vi "level_control_tank.vi"() -> ()   [LabVIEW 2022 SP3]
uses:
  <vilib>/Instr/_visa.llb/VISA Configure Serial Port (Instr).vi
panel:
  out "Tank":i16(slide) scale=0.0..4000.0
  in  "stop":bool
  in  "Baudrate":string(combo)
  in  "Connect":bool
  in  "VISA resource name":refnum<visa-resource-name>
  in  "Slide":i16(slide) scale=0.0..4000.0
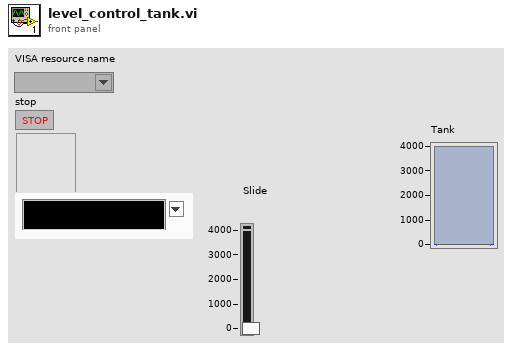
[diagram p1: front panel]
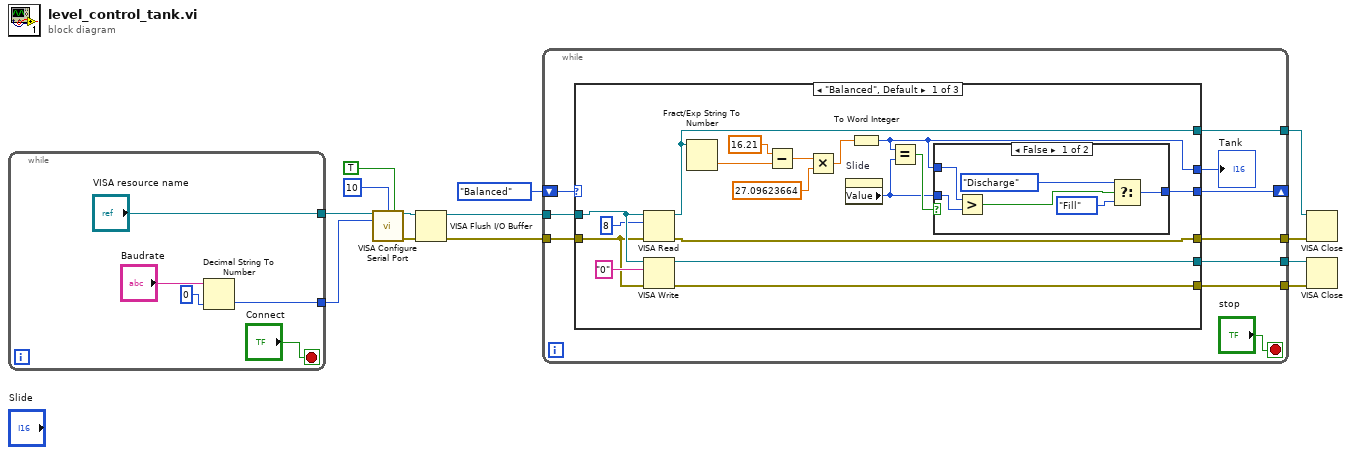
[diagram p0: block diagram]
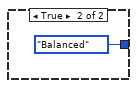
[diagram p2: hidden frame]
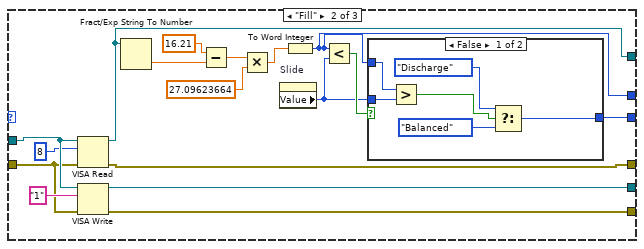
[diagram p3: hidden frame]
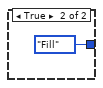
[diagram p4: hidden frame]
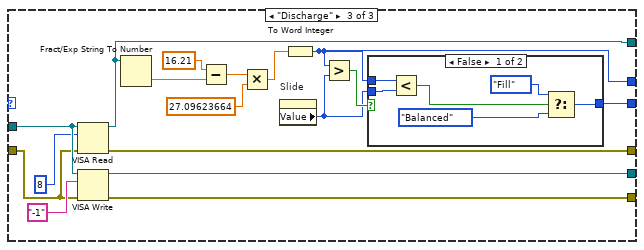
[diagram p5: hidden frame]
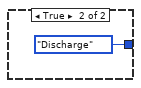
[diagram p6: hidden frame]
diagram:
  n1 = while {
    tunnel: ["VISA resource name"] -> w10
    tunnel: [w17] -> w11
    stop <- "Connect" stop-if-true
    n2 = Decimal String To Number(string="Baudrate", default (0L)=0 ("default (0 I32)")) -> (number=w17:i32)  [unwired: 1 in, 1 out]
  }
  n3 = call-poly "VISA Configure Serial Port"("VISA resource name"=w10, "termination char\n(0xA = '\\n' = LF)"=u8 10 ("termination char\n(0xA = '\\n' = LF)"), "Enable Termination\nChar (T)"=TRUE ("Enable Termination\nChar (T)"), "baud rate (9600)"=w11) -> ("VISA resource name out"=w9:refnum<visa-resource-name>, "error out"=w8:errorcluster)  [unwired: 10 in]
  n4 = VISA Flush I/O Buffer(VISA resource name=w9, error in (no error)=w8) -> (VISA resource name out=w6:refnum<visa-resource-name>, error out=w5:errorcluster)  [unwired: 1 in]
  n5 = while {
    shift-right: [w20] -> _
    shift-left: enum16{"Balanced", "Fill", "Discharge"}."Balanced" -> [w28]
    tunnel: w6 -> [w27]
    tunnel: w5 -> [w26]
    tunnel: [w25] -> w4
    tunnel: [w24] -> w3
    tunnel: [w22] -> w2
    tunnel: [w21] -> w1
    stop <- "stop" stop-if-true
    n6 = case shown="\"Balanced\", Default" w28 {
      tunnel: w27 -> [w41 w67 w91]
      tunnel: w26 -> [w40 w66 w90]
      tunnel: [w44 w65 w89] -> w25
      tunnel: [w43 w64 w88] -> w24
      tunnel: [w32 w55 w80] -> w22
      tunnel: [w42 w63 w87] -> w21
      tunnel: [w39 w62 w86] -> w20
      tunnel: [w29 w53 w77] -> w19
      frame "Balanced", Default {
        n7 = VISA Read(VISA resource name=w41, byte count=u32 8, error in (no error)=w40) -> (VISA resource name out=w32:refnum<visa-resource-name>, error out=w42:errorcluster)  [unwired: 2 out]
        n8 = VISA Write(VISA resource name=w41, write buffer="0", error in (no error)=w40) -> (VISA resource name out=w44:refnum<visa-resource-name>, error out=w43:errorcluster)  [unwired: 1 out]
        n9 = Fract/Exp String To Number(string=w32) -> (number=w35:dbl)  [unwired: 3 in, 1 out]
        n10 = Subtract(x=16.21, y=w35) -> (x-y=w33:dbl)
        n11 = Multiply(x=w33, y=27.09623664) -> (x*y=w31:dbl)
        n12 = property on="Slide" class="Slide (strict)"() -> ("Value"=w30:i16)  [unwired: 2 in, 2 out]
        n13 = To Word Integer(number=w31) -> (16bit integer=w29:i16)
        n14 = Equal?(x=w29, y=w30) -> (x = y?=w38:bool)
        n15 = case shown="False" w38 {
          tunnel: [w48 enum16{"Balanced", "Fill", "Discharge"}."Balanced"] -> w39
          tunnel: w29 -> [w47 _]
          tunnel: w30 -> [w46 _]
          frame False {
            n16 = Greater?(x=w47, y=w46) -> (0:w51:bool)
            n17 = Select(t=enum16{"Balanced", "Fill", "Discharge"}."Discharge", s=w51, f=enum16{"Balanced", "Fill", "Discharge"}."Fill") -> (s? t:f=w48:enum16{"Balanced", "Fill", "Discharge"})
          }
          frame True {
          }
        }
      }
      frame "Fill" {
        n18 = VISA Read(VISA resource name=w67, byte count=u32 8, error in (no error)=w66) -> (VISA resource name out=w55:refnum<visa-resource-name>, error out=w63:errorcluster)  [unwired: 2 out]
        n19 = VISA Write(VISA resource name=w67, write buffer="1", error in (no error)=w66) -> (VISA resource name out=w65:refnum<visa-resource-name>, error out=w64:errorcluster)  [unwired: 1 out]
        n20 = Fract/Exp String To Number(string=w55) -> (number=w59:dbl)  [unwired: 3 in, 1 out]
        n21 = Subtract(x=16.21, y=w59) -> (x-y=w57:dbl)
        n22 = Multiply(x=w57, y=27.09623664) -> (x*y=w56:dbl)
        n23 = property on="Slide" class="Slide (strict)"() -> ("Value"=w54:i16)  [unwired: 2 in, 2 out]
        n24 = To Word Integer(number=w56) -> (16bit integer=w53:i16)
        n25 = Less?(x=w53, y=w54) -> (x < y?=w68:bool)
        n26 = case shown="False" w68 {
          tunnel: [w72 enum16{"Balanced", "Fill", "Discharge"}."Fill"] -> w62
          tunnel: w53 -> [w71 _]
          tunnel: w54 -> [w70 _]
          frame False {
            n27 = Greater?(x=w71, y=w70) -> (0:w75:bool)
            n28 = Select(t=enum16{"Balanced", "Fill", "Discharge"}."Discharge", s=w75, f=enum16{"Balanced", "Fill", "Discharge"}."Balanced") -> (s? t:f=w72:enum16{"Balanced", "Fill", "Discharge"})
          }
          frame True {
          }
        }
      }
      frame "Discharge" {
        n29 = VISA Read(VISA resource name=w91, byte count=u32 8, error in (no error)=w90) -> (VISA resource name out=w80:refnum<visa-resource-name>, error out=w87:errorcluster)  [unwired: 2 out]
        n30 = VISA Write(VISA resource name=w91, write buffer="-1", error in (no error)=w90) -> (VISA resource name out=w89:refnum<visa-resource-name>, error out=w88:errorcluster)  [unwired: 1 out]
        n31 = Fract/Exp String To Number(string=w80) -> (number=w83:dbl)  [unwired: 3 in, 1 out]
        n32 = Subtract(x=16.21, y=w83) -> (x-y=w82:dbl)
        n33 = Multiply(x=w82, y=27.09623664) -> (x*y=w81:dbl)
        n34 = property on="Slide" class="Slide (strict)"() -> ("Value"=w78:i16)  [unwired: 2 in, 2 out]
        n35 = To Word Integer(number=w81) -> (16bit integer=w77:i16)
        n36 = Greater?(x=w77, y=w78) -> (0:w92:bool)
        n37 = case shown="False" w92 {
          tunnel: [w96 enum16{"Balanced", "Fill", "Discharge"}."Discharge"] -> w86
          tunnel: w77 -> [w95 _]
          tunnel: w78 -> [w94 _]
          frame False {
            n38 = Less?(x=w95, y=w94) -> (x < y?=w99:bool)
            n39 = Select(t=enum16{"Balanced", "Fill", "Discharge"}."Fill", s=w99, f=enum16{"Balanced", "Fill", "Discharge"}."Balanced") -> (s? t:f=w96:enum16{"Balanced", "Fill", "Discharge"})
          }
          frame True {
          }
        }
      }
    }
    "Tank" <- w19
  }
  n40 = VISA Close(VISA resource name=w2, error in (no error)=w1) -> ()  [unwired: 1 out]
  n41 = VISA Close(VISA resource name=w4, error in (no error)=w3) -> ()  [unwired: 1 out]
